vi "Open.vi"(8 "error in (no error)":errorcluster, 11 "BiStableShutter in":refnum<class "BiStableShutter.lvclass">) -> (0 "error out":errorcluster, 3 "BiStableShutter out":refnum<class "BiStableShutter.lvclass">)   [LabVIEW 2016, in "BiStableShutter.lvclass"]
uses:
  BiStableShutter.lvclass
  Shutter.lvclass
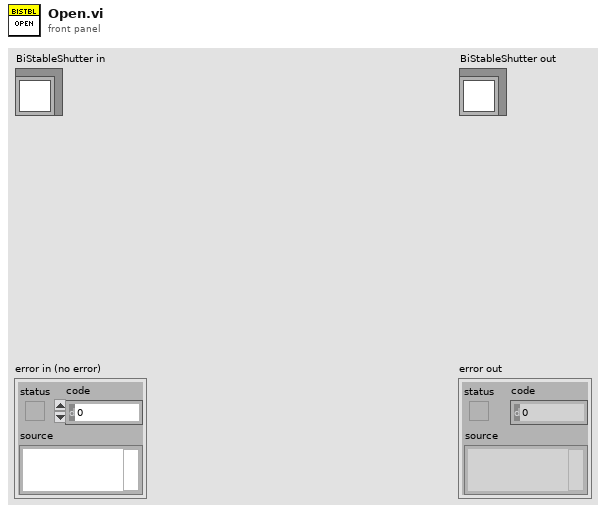
[diagram p1: front panel]
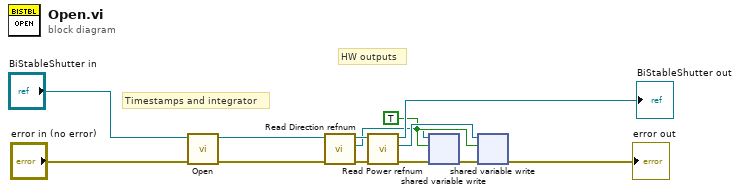
[diagram p0: block diagram]
diagram:
  w6 = TRUE
  # "HW outputs"
  # "Timestamps and integrator"
  n1 = call-parent "Open.vi"("error in (no error)"="error in (no error)", "Shutter in"="BiStableShutter in") -> ("error out"=w2:errorcluster, "Shutter out"=w1:refnum<class "BiStableShutter.lvclass">)  [unwired: 8 in]
  n2 = call-dynamic "Read Direction refnum.vi"("error in (no error)"=w2, "BiStableShutter in"=w1) -> ("error out"=w8:errorcluster, "Direction refnum"=w5:refnum<k21>, "BiStableShutter out"=w9:refnum<class "BiStableShutter.lvclass">)  [unwired: 7 in]
  n3 = call-dynamic "Read Power refnum.vi"("error in (no error)"=w8, "BiStableShutter in"=w9) -> ("error out"=w4:errorcluster, "Power refnum"=w7:refnum<k21>, "BiStableShutter out"=→"BiStableShutter out":refnum<class "BiStableShutter.lvclass">)  [unwired: 7 in]
  n4 = shared-variable-write(w5, w4, w6) -> (w3:errorcluster)  [unwired: 1 out]
  n5 = shared-variable-write(w7, w3, w6) -> (→"error out":errorcluster)  [unwired: 1 out]
